vi "Logging Get by Name.vi"(1 "Name":string, 2 "Entries":T1[](array[typedef])) -> (0 "Entry":T1)   [LabVIEW 2012, in "femtoRoboLib.lvlib"]
uses:
  Log Entry.ctl
  Log Value Type.ctl
  Log Value Cluster.ctl
  femtoRoboLib.lvlib
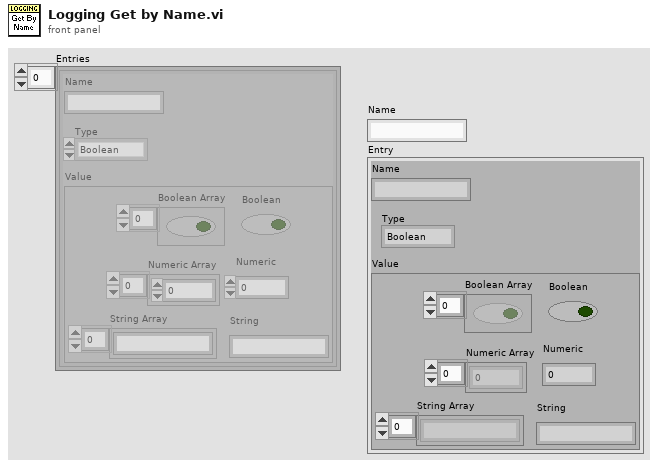
[diagram p1: front panel]
types:
  T1 = typedef "femtoRoboLib.lvlib/Log Entry.ctl" = cluster{"Name":string, "Type":T2, "Value":T3}
  T2 = typedef "femtoRoboLib.lvlib/Log Value Type.ctl" = enum16{"Boolean", "Numeric", "String", "Boolean Array", "Numeric Array", "String Array"}
  T3 = typedef "femtoRoboLib.lvlib/Log Value Cluster.ctl" = cluster{"Boolean Array":bool[], "Boolean":bool, "Numeric Array":dbl[], "Numeric":dbl, "String Array":string[], "String":string}
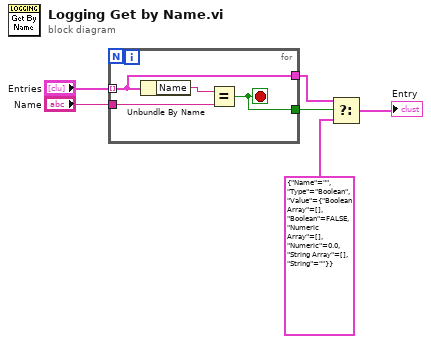
[diagram p0: block diagram]
diagram:
  n1 = for {
    tunnel: "Entries" -> [w9] mode=indexing
    tunnel: "Name" -> [w10]
    tunnel: [w9] -> w4
    tunnel: [w8] -> w5
    stop <- w8 stop-if-true
    n2 = Unbundle By Name(w9) -> ("Name"=w7:string)
    n3 = Equal?(x=w7, y=w10) -> (x = y?=w8:bool)
  }
  n4 = Select(t=w4, s=w5, f=T1 {"Name"="", "Type"=enum."Boolean", "Value"={"Boolean Array"=[], "Boolean"=FALSE, "Numeric Array"=[], "Numeric"=0.0, "String Array"=[], "String"=""}}) -> (s? t:f=→"Entry":T1)
